vi "rgpna.vi"() -> ()   [LabVIEW 2010]
uses:
  <vilib>/Utility/error.llb/DialogType.ctl
  <vilib>/measure/maspectr.llb/FFT Power Spectrum and PSD for 1 Chan.vi
  <vilib>/Platform/browser.llb/Open URL in Default Browser (string).vi
  user32.dll
  <vilib>/measure/NI_MAPro.lvlib
panel:
  in  "Tab Control":enum32{"View/Edit", "History", "List", "Graph"}(tab)
  in  "String":string
  out "Table":string[][](table)
  in  "Tree":string(tree)
  out "Waveform Graph":cluster{"f0":dbl, "df":dbl, "magnitude":dbl[]}[](graph) caption="-----------------------------------------------------------------------------------"
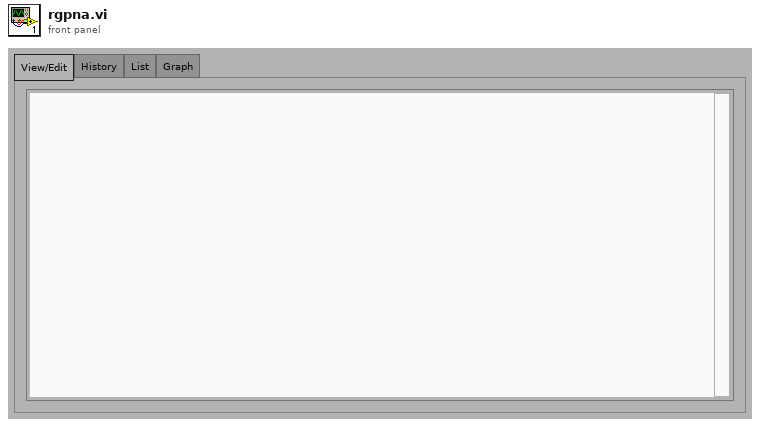
[diagram p1: front panel]
types:
  T1 = typedef "DialogType.ctl" = u16
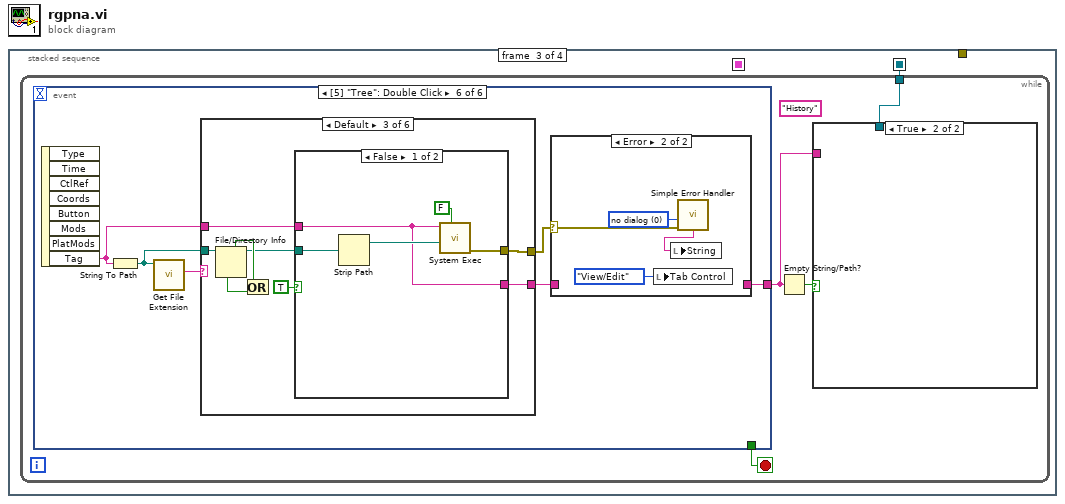
[diagram p0: block diagram]
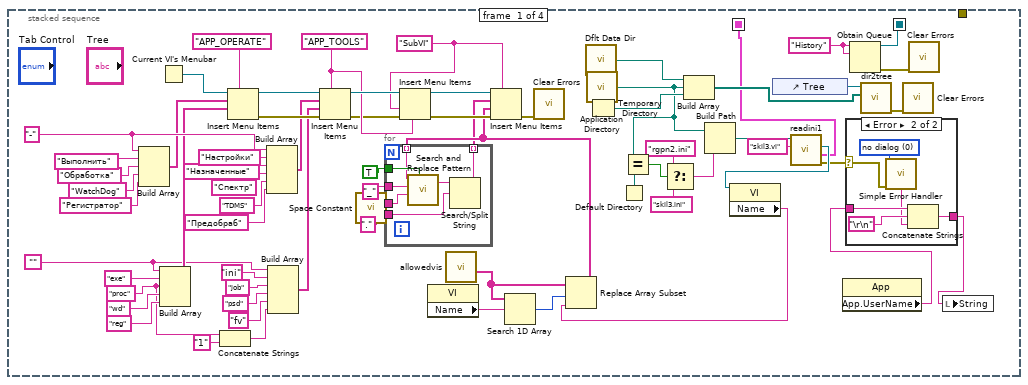
[diagram p2: hidden frame]
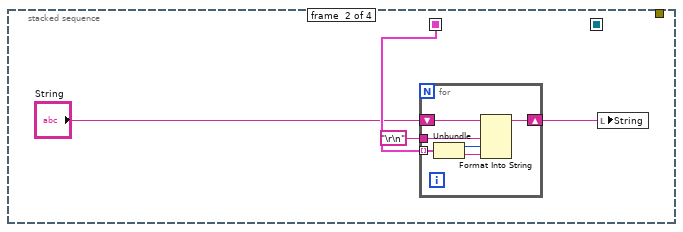
[diagram p4: hidden frame]
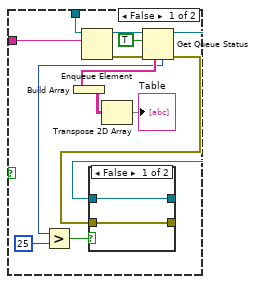
[diagram p5: hidden frame]
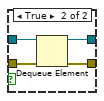
[diagram p6: hidden frame]
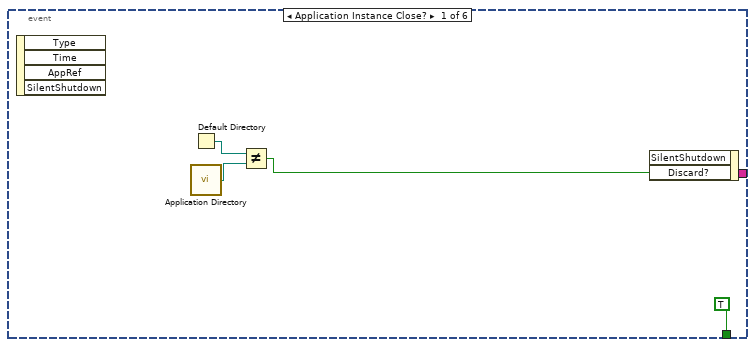
[diagram p7: hidden frame]
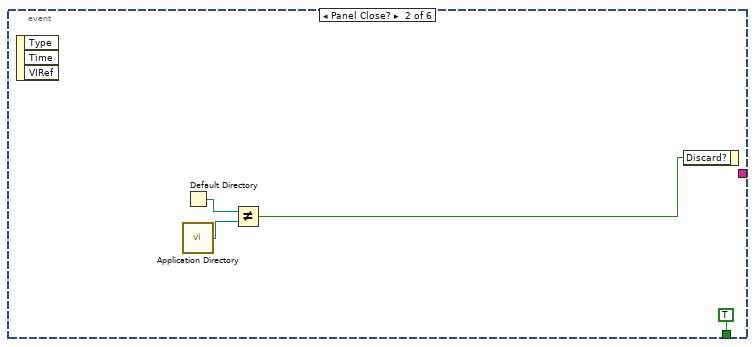
[diagram p8: hidden frame]
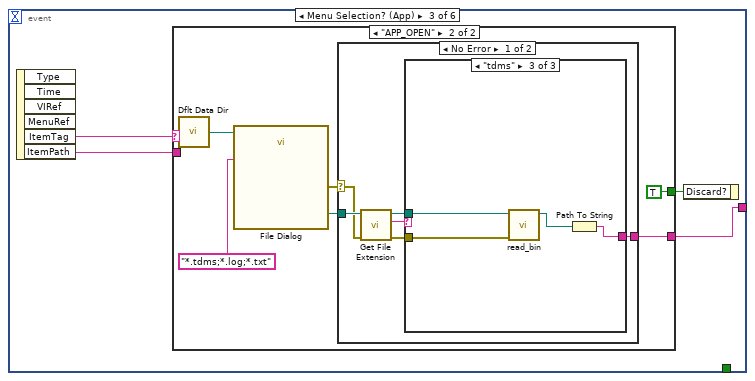
[diagram p9: hidden frame]
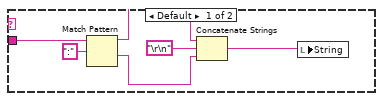
[diagram p10: hidden frame]
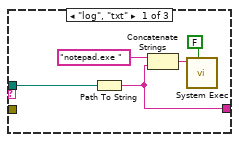
[diagram p11: hidden frame]
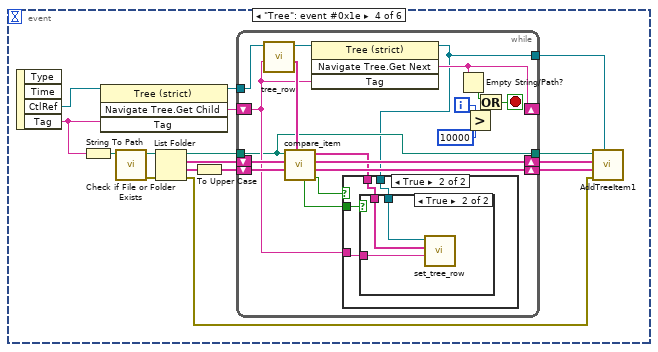
[diagram p14: hidden frame]
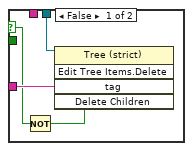
[diagram p15: hidden frame]
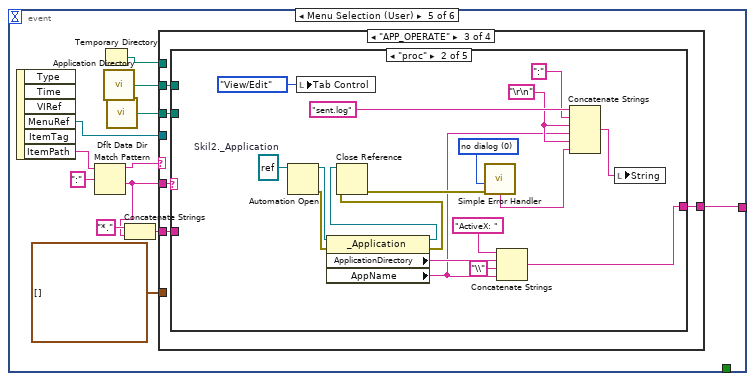
[diagram p17: hidden frame]
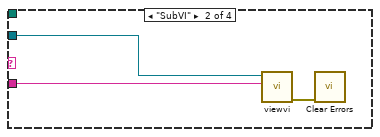
[diagram p19: hidden frame]
diagram:
  n1 = stacked-sequence {
    seq-local: [w51 _ _ _] -> [_ _ w92 w457]
    seq-local: [w13 _ _ _] -> [_ w85 _ _]
    tunnel: [_ _ _ w455] -> _
    frame #0 {
      w43 = "SubVI"
      w3 = "proc" ("element")
      w53 = "History" ("name (unnamed)")
      w54 = ""
      w62 = "-"
      w44 = "APP_TOOLS" ("menu tag")
      n2 = Build Array(w62, "Выполнить", "Обработка", "WatchDog" ("element"), "Регистратор" ("element")) -> (w57:string[])
      n3 = Current VI's Menubar() -> (w67:refnum<k9>)
      n4 = Build Array(w54, "exe", w3, "wd" ("element"), "reg" ("element")) -> (w58:string[])
      n5 = Concatenate Strings(w3, "1" ("string")) -> (w1:string)
      n6 = Insert Menu Items(5:"APP_OPERATE", 7:w58, 8:w57, 9:w67) -> (0:w65:errorcluster, 3:w64:refnum<k9>)  [unwired: 2 in, 1 out]
      n7 = Build Array(w62, "Настройки", "Назначенные" ("element"), "Спектр" ("element"), "TDMS" ("element"), "Предобраб" ("element")) -> (w55:string[])
      n8 = Build Array(w54, "ini", "job" ("element"), "psd" ("element"), "fv" ("element"), w1) -> (w56:string[])
      n9 = Insert Menu Items(5:w44, 6:w65, 7:w56, 8:w55, 9:w64) -> (0:w41:errorcluster, 3:w45:refnum<k9>)  [unwired: 1 in, 1 out]
      n10 = call <vilib>:"Space Constant.vi"() -> ("String"=w15:string)
      n11 = Insert Menu Items(4:w44, 6:w41, 7:w43, 9:w45) -> (0:w40:errorcluster, 3:w42:refnum<k9>)  [unwired: 2 in, 1 out]
      n12 = property class="VI"() -> ("Name"=w29:string)  [unwired: 2 in, 2 out]
      n13 = call "allowedvis.vi"() -> ("AllowedVis"=w38:string[])  [unwired: 6 in, 1 out]
      n14 = Search 1D Array(1D array=w38, element=w29) -> (index of element=w32:i32)  [unwired: 1 in]
      n15 = call <vilib>:"Dflt Data Dir.vi"() -> ("App:Default Data Directory"=w37:path)
      n16 = call <vilib>:"Application Directory.vi"() -> ("Application Directory"=w28:path)
      n17 = Temporary Directory() -> (w36:path)
      n18 = Default Directory() -> (w27:path)
      n19 = Equal?(x=w28, y=w27) -> (x = y?=w26:bool)
      n20 = Select(t="rgpn2.ini" ("name or relative path"), s=w26, f="skil3.ini") -> (s? t:f=w24:string)
      n21 = Build Array(w37, w28, w36) -> (w35:path[])
      n22 = Build Path(base path=w28, name or relative path=w24) -> (appended path=w34:path)
      n23 = control-ref of="Tree"() -> (w52:refnum<vi>)
      n24 = call "readini1.vi"("section"="skil3.vi", "configuration file path"=w34) -> ("error out"=w22:errorcluster, "Dev_Gr"=w13:cluster{"DevNo":i32, "Group":string}[], "global2vi_ref"=w31:refnum<vi>)  [unwired: 2 in, 1 out]
      n25 = property class="VI"(reference=w31) -> ("Name"=w30:string)  [unwired: 1 in, 2 out]
      n26 = Replace Array Subset(array=w38, new element=w30, index=w32) -> (w19:string[])
      n27 = for {
        tunnel: "_" ("regular expression (\"\")") -> [w74]
        tunnel: TRUE ("replace all? (F)") -> [w73]
        tunnel: w19 -> [w72] mode=indexing
        tunnel: [w69] -> w18 mode=indexing
        tunnel: w15 -> [w71]
        tunnel: "." ("regular expression (\"\")") -> [w68]
        n28 = call <vilib>:"Search and Replace Pattern.vi"("string"=w72, "regular expression (\"\")"=w74, "replace string (\"\")"=w71, "replace all? (F)"=w73) -> ("result string"=w70:string)  [unwired: 1 in, 1 out]
        n29 = Search/Split String(string=w70, search string/char (-)=w68) -> (substring before match=w69:string)  [unwired: 1 in, 2 out]
      }
      n30 = Insert Menu Items(5:w43, 6:w40, 7:w19, 8:w18, 9:w42) -> (0:w39:errorcluster)  [unwired: 1 in, 2 out]
      n31 = call <vilib>:"Clear Errors.vi"("error in (no error)"=w39) -> ()  [unwired: 6 in, 1 out]
      n32 = property class="App"() -> ("App.UserName"=w12:string)  [unwired: 2 in, 2 out]
      n33 = case shown="Error" w22 {
        selector: w22 -> [_ w80]
        tunnel: w12 -> [w75 w78]
        tunnel: [w75 w79] -> w11
        frame No Error {
        }
        frame Error {
          w81 = T1 0 items=["no dialog", "OK message", "continue or stop message", "OK message + warnings", "continue/stop + warnings"] ("type of dialog (OK msg:1)")
          n34 = call <vilib>:"Simple Error Handler.vi"("type of dialog (OK msg:1)"=w81, "error in (no error)"=w80) -> ("message"=w76:string)  [unwired: 3 in, 4 out]
          n35 = Concatenate Strings(w78, "\r\n", w76) -> (w79:string)
        }
      }
      n36 = Obtain Queue(name (unnamed)=w53, element data type=w53) -> (queue out=w51:refnum<queue>, error out=w50:errorcluster)  [unwired: 3 in, 1 out]
      n37 = call "dir2tree.vi"("Dirs"=w35, "Tree"=w52) -> ("error out"=w49:errorcluster)  [unwired: 4 in, 1 out]
      n38 = call <vilib>:"Clear Errors.vi"("error in (no error)"=w49) -> ()  [unwired: 6 in, 1 out]
      n39 = call <vilib>:"Clear Errors.vi"("error in (no error)"=w50) -> ()  [unwired: 6 in, 1 out]
      n40 = local write "String"(w11) -> ()
    }
    frame #1 {
      n41 = for {
        tunnel: w85 -> [w91] mode=indexing
        shift-right: [w87] -> w83
        shift-left: "String" -> [w90]
        tunnel: "\r\n" -> [w86]
        n42 = Unbundle(w91) -> ("DevNo"=w89:i32, "Group"=w88:string)
        n43 = Format Into String(initial string=w90, w86, w89, w88) -> (resulting string=w87:string)  [unwired: 2 in, 1 out]
      }
      n44 = local write "String"(w83) -> ()
    }
    frame #2 {
      n45 = while {
        tunnel: w92 -> [w93]
        stop <- w96 stop-if-true
        (unwired) "History" ("name (unnamed)")
        n46 = event shown="[5] \"Tree\": Double Click" {
          selector: _ -> [_ _ _ _ _ _]
          dyn-events: _ -> [_ _ _ _ _ _]
          timeout: _ -> [_ _ _ _ _ _]
          tunnel: [TRUE ("SilentShutdown") TRUE ("SilentShutdown") _ _ _ _] -> w96
          tunnel: [_ _ w124 _ w204 w403] -> w94
          event Application Instance Close? {
            n47 = event-data() -> ()  [unwired: 1 in, 4 out]
            n48 = Default Directory() -> (w119:path)
            n49 = call <vilib>:"Application Directory.vi"() -> ("Application Directory"=w118:path)
            n50 = Not Equal?(x=w119, y=w118) -> (x != y?=w117:bool)
            n51 = event-data("Discard?"=w117) -> ()  [unwired: 2 in, 1 out]
          }
          event Panel Close? {
            n52 = event-data() -> ()  [unwired: 1 in, 3 out]
            n53 = Default Directory() -> (w123:path)
            n54 = call <vilib>:"Application Directory.vi"() -> ("Application Directory"=w122:path)
            n55 = Not Equal?(x=w123, y=w122) -> (x != y?=w121:bool)
            n56 = event-data("Discard?"=w121) -> ()  [unwired: 1 in, 1 out]
          }
          event Menu Selection? (App) {
            n57 = event-data() -> ("ItemTag"=w127:string, "ItemPath"=w125:string)  [unwired: 1 in, 4 out]
            n58 = case shown="\"APP_OPEN\"" w127 {
              tunnel: [_ TRUE ("Discard?")] -> w126
              tunnel: w125 -> [w133 _]
              tunnel: [_ w134] -> w124
              frame Default {
                n59 = Match Pattern(string=w133, regular expression=":") -> (before substring=w131:string, after substring=w130:string)  [unwired: 1 in, 2 out]
                n60 = Concatenate Strings(w131, "\r\n", w130) -> (w128:string)
                n61 = local write "String"(w128) -> ()
              }
              frame "APP_OPEN" {
                n62 = call <vilib>:"Dflt Data Dir.vi"() -> ("App:Default Data Directory"=w138:path)
                n63 = call "File Dialog"("start path"=w138, "pattern (all files)"="*.tdms;*.log;*.txt") -> ("selected path"=w136:path, "error out"=w135:errorcluster)  [unwired: 10 in, 2 out]
                n64 = case shown="No Error" w135 {
                  selector: w135 -> [w141 _]
                  tunnel: w136 -> [w145 _]
                  tunnel: [w140 _] -> w134
                  frame No Error {
                    n65 = call <vilib>:"Get File Extension.vi"("error in (no error)"=w141, "file"=w145) -> ("error out"=w143:errorcluster, "lowercase file extension"=w144:string, "dup file"=w142:path)  [unwired: 6 in, 1 out]
                    n66 = case shown="\"tdms\"" w144 {
                      tunnel: w143 -> [_ _ w154]
                      tunnel: w142 -> [w147 _ w153]
                      tunnel: [w146 _ w151] -> w140
                      frame "log", "txt" {
                        n67 = Path To String(path=w147) -> (string=w146:string)
                        n68 = Concatenate Strings("notepad.exe " ("string"), w146) -> (w149:string)
                        n69 = call <vilib>:"System Exec.vi"("wait until completion? (T)"=FALSE, "command line"=w149) -> ()  [unwired: 6 in, 4 out]
                      }
                      frame Default {
                      }
                      frame "tdms" {
                        n70 = call "read_bin.vi"("error in"=w154, "datalog path"=w153) -> ("new file path"=w152:path)  [unwired: 2 in, 3 out]
                        n71 = Path To String(path=w152) -> (string=w151:string)
                      }
                    }
                  }
                  frame Error {
                  }
                }
              }
            }
            n72 = event-data("Discard?"=w126) -> ()  [unwired: 1 in, 1 out]
          }
          event "Tree": event #0x1e {
            n73 = event-data() -> ("CtlRef"=w170:refnum<vi>, "Tag"=w160:string)  [unwired: 1 in, 2 out]
            n74 = String To Path(string=w160) -> (path=w167:path)
            n75 = invoke class="Tree (strict)" method="Navigate Tree.Get Child"(reference=w170, "Tag"=w160) -> (reference out=w169:refnum<vi>, "Navigate Tree:Get Child"=w168:string)  [unwired: 2 in, 2 out]
            n76 = call <vilib>:"Check if File or Folder Exists.vi"("path"=w167) -> ("error out"=w166:errorcluster, "dup path"=w165:path)  [unwired: 8 in, 1 out]
            n77 = List Folder(path=w165, error in=w166) -> (path out=w163:path, filenames=w162:string[], folder names=w164:string[], error out=w155:errorcluster)  [unwired: 2 in]
            n78 = To Upper Case(1:w164) -> (0:w161:string[])
            n79 = while {
              tunnel: w169 -> [w184]
              tunnel: w163 -> [w172]
              shift-right: [w186] -> w158
              shift-left: w161 -> [w187]
              shift-right: [w185] -> w159
              shift-left: w162 -> [w188]
              shift-right: [w182] -> _
              shift-left: w168 -> [w175]
              tunnel: [w172] -> w157
              tunnel: [w171] -> w156
              i -> [w181]
              stop <- w177 stop-if-true
              n80 = call "tree_row.vi"("Tag"=w175, "CtlRef"=w184) -> ("Row"=w189:string[], "CtlRef 2"=w183:refnum<vi>)  [unwired: 3 in, 1 out]
              n81 = call "compare_item.vi"("item"=w189, "folders"=w187, "filenames"=w188, "start path"=w172) -> ("exist"=w176:bool, "folders 2"=w186:string[], "filenames 2"=w185:string[], "item 2"=w173:string[], "modified"=w174:bool)  [unwired: 1 in]
              n82 = invoke class="Tree (strict)" method="Navigate Tree.Get Next"(reference=w183, "Tag"=w175) -> (reference out=w171:refnum<vi>, "Navigate Tree:Get Next Item"=w182:string)  [unwired: 2 in, 2 out]
              n83 = case shown="True" w176 {
                selector: w176 -> [w190 _]
                tunnel: w171 -> [w193 w196]
                tunnel: w175 -> [w192 w195]
                tunnel: w174 -> [_ w197]
                tunnel: w173 -> [_ w194]
                frame False {
                  n84 = Not(x=w190) -> (.not. x?=w191:bool)
                  n85 = invoke class="Tree (strict)" method="Edit Tree Items.Delete"(reference=w193, "tag"=w192, "Delete Children"=w191) -> ()  [unwired: 2 in, 5 out]
                }
                frame True {
                  n86 = case shown="True" w197 {
                    tunnel: w196 -> [_ w200]
                    tunnel: w195 -> [_ w199]
                    tunnel: w194 -> [_ w198]
                    frame False {
                      # "do nothing"
                    }
                    frame True {
                      n87 = call "set_tree_row.vi"("Tag"=w199, "Row"=w198, "CtlRef"=w200) -> ()  [unwired: 3 in, 2 out]
                    }
                  }
                }
              }
              n88 = Empty String/Path?(string/path=w182) -> (empty?=w179:bool)
              n89 = Greater?(x=w181, y=10000) -> (0:w178:bool)
              n90 = Or(x=w179, y=w178) -> (x .or. y?=w177:bool)
            }
            n91 = call "AddTreeItem1.vi"("CtlRef 2"=w156, "error in"=w155, "folder names"=w158, "filenames"=w159, "path"=w157) -> ()  [unwired: 1 in, 4 out]
          }
          event Menu Selection (User) {
            n92 = event-data() -> ("MenuRef"=w202:refnum<k9>, "ItemPath"=w211:string)  [unwired: 1 in, 4 out]
            n93 = Match Pattern(string=w211, regular expression=":") -> (before substring=w210:string, after substring=w208:string)  [unwired: 1 in, 2 out]
            n94 = Temporary Directory() -> (w205:path)
            n95 = call <vilib>:"Application Directory.vi"() -> ("Application Directory"=w206:path)
            n96 = call <vilib>:"Dflt Data Dir.vi"() -> ("App:Default Data Directory"=w203:path)
            n97 = Concatenate Strings("*." ("string"), w208) -> (w207:string)
            n98 = case shown="\"APP_OPERATE\"" w210 {
              tunnel: w208 -> [_ w215 w220 w302]
              tunnel: w207 -> [_ _ w219 w301]
              tunnel: w206 -> [_ _ w218 w300]
              tunnel: w205 -> [_ _ _ _]
              tunnel: [_ _ w217 w299] -> w204
              tunnel: w203 -> [_ _ w216 w297]
              tunnel: w202 -> [_ w214 _ _]
              tunnel: waveform(i16)[] [] ("Waveform Graph") -> [_ _ _ w298]
              frame Default {
              }
              frame "SubVI" {
                n99 = call "viewvi.vi"("item tag"=w215, "menu reference"=w214) -> ("error out"=w213:errorcluster)  [unwired: 5 in]
                n100 = call <vilib>:"Clear Errors.vi"("error in (no error)"=w213) -> ()  [unwired: 6 in, 1 out]
              }
              frame "APP_OPERATE" {
                n101 = case shown="\"proc\"" w220 {
                  tunnel: w219 -> [_ _ _ w256 _]
                  tunnel: w218 -> [_ _ _ w255 _]
                  tunnel: [_ w228 w246 w254 w264] -> w217
                  tunnel: w216 -> [_ _ _ _ w269]
                  frame Default {
                  }
                  frame "proc" {
                    w232 = "\r\n"
                    w236 = T1 0 items=["no dialog", "OK message", "continue or stop message", "OK message + warnings", "continue/stop + warnings"] ("type of dialog (OK msg:1)")
                    w238 = refnum<k7> refnum  # Skil2._Application
                    n102 = Automation Open(Automation Refnum=w238) -> (Automation Refnum=w230:refnum<k7>, error out=w227:errorcluster)  [unwired: 3 in]
                    n103 = local write "Tab Control"(enum32{"View/Edit", "History", "List", "Graph"}."View/Edit" ("Tab Control")) -> ()
                    n104 = property class="_Application"(reference=w230, error in=w227) -> (reference out=w226:refnum<k7>, error out=w225:errorcluster, "ApplicationDirectory"=w229:string, "AppName"=w221:string)
                    n105 = Close Reference(reference=w226, error in (no error)=w225) -> (error out=w222:errorcluster)
                    n106 = call <vilib>:"Simple Error Handler.vi"("type of dialog (OK msg:1)"=w236, "error in (no error)"=w222) -> ("message"=w231:string)  [unwired: 3 in, 4 out]
                    n107 = Concatenate Strings("ActiveX: " ("string"), w229, "\\" ("string"), w221) -> (w228:string)
                    n108 = Concatenate Strings("sent.log" ("name or relative path"), ":" ("string"), w232, w221, w232, w231) -> (w234:string)
                    n109 = local write "String"(w234) -> ()
                  }
                  frame "reg" {
                    w249 = refnum<k7> refnum  # Rgpn2._Application
                    n110 = Automation Open(Automation Refnum=w249) -> (Automation Refnum=w248:refnum<k7>, error out=w245:errorcluster)  [unwired: 3 in]
                    n111 = property class="_Application"(reference=w248, error in=w245) -> (reference out=w244:refnum<k7>, error out=w243:errorcluster, "ApplicationDirectory"=w247:string, "AppName"=w241:string)
                    n112 = Close Reference(reference=w244, error in (no error)=w243) -> (error out=w239:errorcluster)
                    n113 = case shown="Error" w239 {
                      selector: w239 -> [_ w251]
                      frame No Error {
                      }
                      frame Error {
                        w253 = T1 0 items=["no dialog", "OK message", "continue or stop message", "OK message + warnings", "continue/stop + warnings"] ("type of dialog (OK msg:1)")
                        n114 = call <vilib>:"Simple Error Handler.vi"("type of dialog (OK msg:1)"=w253, "error in (no error)"=w251) -> ("message"=w252:string)  [unwired: 3 in, 4 out]
                        n115 = local write "Tab Control"(enum32{"View/Edit", "History", "List", "Graph"}."View/Edit" ("Tab Control")) -> ()
                        n116 = local write "String"(w252) -> ()
                      }
                    }
                    n117 = Concatenate Strings("ActiveX: " ("string"), w247, "\\" ("string"), w241) -> (w246:string)
                  }
                  frame "exe" {
                    n118 = call "File Dialog2"("start path"=w255, "pattern (all files)"=w256) -> ("selected path"=w257:path, "error out"=w258:errorcluster)  [unwired: 10 in, 2 out]
                    n119 = case shown="No Error" w258 {
                      tunnel: w255 -> [w262 _]
                      tunnel: w257 -> [w261 _]
                      tunnel: [w259 _] -> w254
                      frame No Error {
                        n120 = Path To String(path=w261) -> (string=w259:string)
                        n121 = call <vilib>:"System Exec.vi"("wait until completion? (T)"=FALSE, "working directory"=w262, "command line"=w259) -> ("error out"=w260:errorcluster)  [unwired: 5 in, 3 out]
                        n122 = call <vilib>:"Clear Errors.vi"("error in (no error)"=w260) -> ()  [unwired: 6 in, 1 out]
                      }
                      frame Error {
                      }
                    }
                  }
                  frame "wd" {
                    w267 = "wd.log" ("name or relative path")
                    w264 = "schtasks /run /tn \"watchdog\"" ("command line")
                    n123 = Build Path(base path=w269, name or relative path=w267) -> (appended path=w268:path)
                    n124 = local write "Tab Control"(enum32{"View/Edit", "History", "List", "Graph"}."View/Edit" ("Tab Control")) -> ()
                    n125 = call <vilib>:"System Exec.vi"("run minimized? (F)"=TRUE, "command line"=w264) -> ("error out"=w274:errorcluster, "standard error"=w266:string, "standard output"=w276:string)  [unwired: 6 in, 1 out]
                    n126 = Concatenate Strings(w276, w266) -> (w275:string)
                    n127 = Empty String/Path?(string/path=w266) -> (empty?=w265:bool)
                    n128 = dll-call lib="user32.dll" fn="OemToCharA"(error in=w274, "src"=w275, "dst"=w275) -> (error out=w273:errorcluster, "dst"=w271:string)  [unwired: 4 in, 1 out]
                    n129 = case shown="No Error" w273 {
                      selector: w273 -> [_ w296]
                      tunnel: [w285 w295] -> w272
                      tunnel: w271 -> [w286 _]
                      tunnel: w268 -> [w287 _]
                      tunnel: w267 -> [w280 _]
                      tunnel: w265 -> [w281 _]
                      tunnel: w264 -> [w278 _]
                      frame No Error {
                        w283 = "\r\n"
                        n130 = case shown="True" w281 {
                          tunnel: w287 -> [_ w292]
                          tunnel: [_ w291] -> w282
                          tunnel: [_ w290] -> _
                          tunnel: w280 -> [_ w289]
                          tunnel: [w288 w289] -> w279
                          tunnel: w278 -> [w288 _]
                          frame False {
                          }
                          frame True {
                            n131 = Read from Text File(file (use dialog)=w292) -> (refnum out=w293:refnum<file>, text=w291:string, error out=w294:errorcluster)  [unwired: 3 in, 1 out]
                            n132 = Close File(refnum=w293, error in=w294) -> (error out=w290:errorcluster)  [unwired: 1 out]
                          }
                        }
                        n133 = Concatenate Strings(w286, w283, w279, ":" ("string"), w283, w282) -> (w285:string)
                      }
                      frame Error {
                        n134 = call <vilib>:"Simple Error Handler.vi"("error in (no error)"=w296) -> ("message"=w295:string)  [unwired: 4 in, 4 out]
                      }
                    }
                    n135 = local write "String"(w272) -> ()
                  }
                }
              }
              frame "APP_TOOLS" {
                n136 = case shown="\"proc1\"" w302 {
                  tunnel: w301 -> [_ _ _ w339 _ _]
                  tunnel: w300 -> [_ _ _ w337 _ _]
                  tunnel: [_ w303 w323 w336 w347 _] -> w299
                  tunnel: w298 -> [_ _ _ _ _ w370]
                  tunnel: w297 -> [_ w312 _ _ _ _]
                  frame Default {
                  }
                  frame "proc1" {
                    n137 = Get Date/Time In Seconds() -> (seconds since 1Jan1904=w307:timestamp)
                    n138 = call "File Dialog5"("start path"=w312, "pattern (all files)"="*.tdms") -> ("selected path"=w309:path, "cancelled"=w310:bool)  [unwired: 10 in, 2 out]
                    n139 = To Double Precision Float(number=w307) -> (double precision float=w308:dbl)
                    n140 = call "to_utc.vi"("Numeric"=w308) -> ("Time Stamp"=w306:timestamp)
                    n141 = case shown="False" w310 {
                      tunnel: w309 -> [w322 _]
                      tunnel: w306 -> [w321 _]
                      tunnel: [w320 _] -> w305
                      tunnel: [w319 _] -> w304
                      frame False {
                        n142 = call "poster1.vi"("last ses time"=w321, "file path"=w322) -> ("error out"=w320:errorcluster, "file dup"=w319:path)  [unwired: 3 in, 1 out]
                      }
                      frame True {
                      }
                    }
                    n143 = case shown="Error" w305 {
                      selector: w305 -> [_ w318]
                      tunnel: w304 -> [w314 _]
                      tunnel: [w313 _] -> w303
                      frame No Error {
                        n144 = Path To String(path=w314) -> (string=w313:string)
                      }
                      frame Error {
                        w317 = T1 0 items=["no dialog", "OK message", "continue or stop message", "OK message + warnings", "continue/stop + warnings"] ("type of dialog (OK msg:1)")
                        n145 = call <vilib>:"Simple Error Handler.vi"("type of dialog (OK msg:1)"=w317, "error in (no error)"=w318) -> ("message"=w316:string)  [unwired: 3 in, 4 out]
                        n146 = local write "Tab Control"(enum32{"View/Edit", "History", "List", "Graph"}."View/Edit" ("Tab Control")) -> ()
                        n147 = local write "String"(w316) -> ()
                      }
                    }
                  }
                  frame "fv" {
                    n148 = call <vilib>:"Dflt Data Dir.vi"() -> ("App:Default Data Directory"=w325:path)
                    n149 = Build Path(base path=w325, name or relative path="Sent") -> (appended path=w324:path)
                    n150 = call "File Dialog4"("start path"=w324, "pattern (all files)"="*.tdms") -> ("selected path"=w330:path, "cancelled"=w327:bool, "error out"=w329:errorcluster)  [unwired: 10 in, 1 out]
                    n151 = case shown="False" w327 {
                      tunnel: [w335 _] -> _
                      tunnel: w330 -> [w334 _]
                      tunnel: w329 -> [w333 _]
                      tunnel: [w331 _] -> w323
                      frame False {
                        n152 = call <vilib>:"TDMS - File Viewer.vi"("error in (no error)"=w333, "file path"=w334) -> ("error out"=w335:errorcluster, "file path out"=w332:path)  [unwired: 4 in]
                        n153 = Path To String(path=w332) -> (string=w331:string)
                      }
                      frame True {
                      }
                    }
                  }
                  frame "ini" {
                    n154 = call "File Dialog3"("start path"=w337, "pattern (all files)"=w339) -> ("selected path"=w338:path, "error out"=w340:errorcluster)  [unwired: 10 in, 2 out]
                    n155 = case shown="No Error" w340 {
                      tunnel: w338 -> [w342 _]
                      tunnel: [w341 _] -> w336
                      frame No Error {
                        n156 = Path To String(path=w342) -> (string=w341:string)
                        n157 = Concatenate Strings("notepad.exe " ("string"), w341) -> (w345:string)
                        n158 = call <vilib>:"System Exec.vi"("wait until completion? (T)"=FALSE, "command line"=w345) -> ("error out"=w343:errorcluster)  [unwired: 6 in, 3 out]
                        n159 = call <vilib>:"Clear Errors.vi"("error in (no error)"=w343) -> ()  [unwired: 6 in, 1 out]
                      }
                      frame Error {
                      }
                    }
                  }
                  frame "job" {
                    (unwired) " /tn watchdog"
                    w347 = "schtasks /query"
                    n160 = call <vilib>:"System Exec.vi"("run minimized? (F)"=TRUE, "command line"=w347) -> ("error out"=w353:errorcluster, "standard error"=w355:string, "standard output"=w356:string)  [unwired: 6 in, 1 out]
                    n161 = local write "Tab Control"(enum32{"View/Edit", "History", "List", "Graph"}."View/Edit" ("Tab Control")) -> ()
                    n162 = Concatenate Strings(w356, w355) -> (w352:string)
                    n163 = dll-call lib="user32.dll" fn="OemToCharA"(error in=w353, "src"=w352, "dst"=w352) -> (error out=w351:errorcluster, "dst"=w350:string)  [unwired: 4 in, 1 out]
                    n164 = case shown="Error" w351 {
                      selector: w351 -> [_ w360]
                      tunnel: [w357 w358] -> w348
                      tunnel: w350 -> [w357 _]
                      frame No Error {
                      }
                      frame Error {
                        w359 = T1 0 items=["no dialog", "OK message", "continue or stop message", "OK message + warnings", "continue/stop + warnings"] ("type of dialog (OK msg:1)")
                        n165 = call <vilib>:"Simple Error Handler.vi"("type of dialog (OK msg:1)"=w359, "error in (no error)"=w360) -> ("message"=w358:string)  [unwired: 3 in, 4 out]
                      }
                    }
                    n166 = local write "String"(w348) -> ()
                  }
                  frame "psd" {
                    n167 = Open VI Reference(vi path="read_bin.vi") -> (vi reference=w381:refnum<vi>, error out=w380:errorcluster)  [unwired: 5 in]
                    n168 = invoke class="VI" method="Ctrl Val.Get"(reference=w381, error in=w380, "Control Name"="Waveform Graph") -> (reference out=w375:refnum<vi>, error out=w377:errorcluster, "Get Control Value Variant"=w378:variant)  [unwired: 1 in, 1 out]
                    n169 = property on="Waveform Graph" class="WFGraph (strict)"("XScale.NameLbl.Text"="Freq" ("X Scale.Name Label.Text"), "YScale.NameLbl.Text"="Mag" ("Y Scale.Name Label.Text"), "XScale.Mapping Mode"=u8 1 ("X Scale.Mapping Mode")) -> ()  [unwired: 2 in, 2 out]
                    n170 = Variant To Data(error in=w377, Variant=w378, type=w370) -> (error out=w365:errorcluster, data=w368:waveform(i16)[])
                    n171 = call "split3.vi"("Array of Waveform In"=w368) -> ("Array of Waveform"=w367:waveform(i16)[])  [unwired: 5 in, 1 out]
                    n172 = Close Reference(reference=w375, error in (no error)=w365) -> (error out=w364:errorcluster)
                    n173 = for {
                      tunnel: w367 -> [w392] mode=indexing
                      tunnel: [w390] -> w366 mode=indexing
                      tunnel: w364 -> [w385]
                      tunnel: [w384] -> w363 mode=indexing
                      i -> [w395]
                      n174 = property on="Waveform Graph" class="WFGraph (strict)"(error in=w385, "Active Plot"=w395) -> (error out=w389:errorcluster, "Plot.Plot Name"=w394:string)  [unwired: 1 in, 1 out]
                      n175 = Get Waveform Attribute(4:w389, 5:w394, 6:"NI_ChannelName", 7:w392) -> (0:w388:errorcluster, 1:w393:string, 3:w396:waveform(i16))  [unwired: 1 out]
                      n176 = property on="Waveform Graph" class="WFGraph (strict)"(error in=w388, "Plot.Plot Name"=w393) -> (error out=w387:errorcluster)  [unwired: 1 in, 1 out]
                      n177 = call "mv2v.vi"("y"=5, "WaveformIn"=w396) -> ("Waveform"=w391:waveform(dbl))  [unwired: 5 in]
                      n178 = call-poly <vilib>:"FFT Power Spectrum and PSD.vi"("error in (no error)"=w387, "time signal"=w391) -> ("error out"=w384:errorcluster, "Power Spectrum / PSD"=w390:cluster{"f0":dbl, "df":dbl, "magnitude":dbl[]})  [unwired: 6 in, 2 out]
                      n179 = Wait (ms)(milliseconds to wait=u32 11) -> ()  [unwired: 1 out]
                    }
                    n180 = control-ref of="Waveform Graph"() -> (w369:refnum<vi>)
                    n181 = Merge Errors(w363) -> (w362:errorcluster)
                    n182 = call "3phColor.vi"("error in (no error)"=w362, "Waveform Graph"=w369) -> ("error out"=w361:errorcluster)  [unwired: 5 in]
                    n183 = case shown="Error" w361 {
                      selector: w361 -> [_ w401]
                      tunnel: w366 -> [w398 _]
                      tunnel: [enum32{"View/Edit", "History", "List", "Graph"}."Graph" ("Tab Control") enum32{"View/Edit", "History", "List", "Graph"}."View/Edit" ("Tab Control")] -> w376
                      frame No Error {
                        "Waveform Graph" <- w398
                      }
                      frame Error {
                        w400 = T1 0 items=["no dialog", "OK message", "continue or stop message", "OK message + warnings", "continue/stop + warnings"] ("type of dialog (OK msg:1)")
                        n184 = call <vilib>:"Simple Error Handler.vi"("type of dialog (OK msg:1)"=w400, "error in (no error)"=w401) -> ("message"=w399:string)  [unwired: 3 in, 4 out]
                        n185 = local write "String"(w399) -> ()
                      }
                    }
                    n186 = local write "Tab Control"(w376) -> ()
                  }
                }
              }
            }
          }
          event "Tree": Double Click {
            n187 = event-data() -> ("Tag"=w407:string)  [unwired: 1 in, 7 out]
            n188 = String To Path(string=w407) -> (path=w406:path)
            n189 = call <vilib>:"Get File Extension.vi"("file"=w406) -> ("lowercase file extension"=w408:string)  [unwired: 7 in, 3 out]
            n190 = case shown="Default" w408 {
              tunnel: w407 -> [w416 w419 w425 w436 w439 w448]
              tunnel: [_ w420 w423 w436 w439 w448] -> w404
              tunnel: w406 -> [w415 _ w429 w437 w443 _]
              tunnel: [w418 w421 w424 w435 w440 w447] -> w405
              frame "cmd", "exe", "vbs" {
                n191 = Strip Path(path=w415) -> (stripped path=w414:path)  [unwired: 1 out]
                n192 = call <vilib>:"System Exec.vi"("wait until completion? (T)"=FALSE, "working directory"=w414, "command line"=w416) -> ("error out"=w418:errorcluster)  [unwired: 5 in, 3 out]
              }
              frame "htm" {
                n193 = call-poly <vilib>:"Open URL in Default Browser.vi"("URL"=w419) -> ("error out"=w421:errorcluster, "URL out"=w420:string)  [unwired: 5 in]
              }
              frame Default {
                n194 = File/Directory Info(path=w429) -> (path out=w426:path, directory=w428:bool, shortcut=w427:bool)  [unwired: 1 in, 4 out]
                n195 = Or(x=w428, y=w427) -> ()  [unwired: 1 out]
                n196 = case shown="False" TRUE {
                  tunnel: w426 -> [w434 _]
                  tunnel: w425 -> [w430 _]
                  tunnel: [w431 _] -> w424
                  tunnel: [w430 _] -> w423
                  frame False {
                    n197 = Strip Path(path=w434) -> (stripped path=w433:path)  [unwired: 1 out]
                    n198 = call <vilib>:"System Exec.vi"("wait until completion? (T)"=FALSE, "working directory"=w433, "command line"=w430) -> ("error out"=w431:errorcluster)  [unwired: 5 in, 3 out]
                  }
                  frame True {
                  }
                }
              }
              frame "tdms" {
                n199 = call "read_bin.vi"("datalog path"=w437) -> ("error out"=w435:errorcluster)  [unwired: 3 in, 3 out]
              }
              frame "dat" {
                n200 = call "convert_dat2tdms.vi"("temporary?"=TRUE, "Path"=w443) -> ("error out"=w438:errorcluster, "New Filel Path"=w441:path)  [unwired: 4 in]
                n201 = case shown="No Error" w438 {
                  selector: w438 -> [_ w446]
                  tunnel: w441 -> [w445 _]
                  tunnel: [w444 w446] -> w440
                  frame No Error {
                    n202 = call "read_bin.vi"("datalog path"=w445) -> ("error out"=w444:errorcluster)  [unwired: 3 in, 3 out]
                  }
                  frame Error {
                  }
                }
              }
              frame "ini", "log", "txt" {
                n203 = Concatenate Strings("notepad.exe " ("string"), w448) -> (w450:string)
                n204 = call <vilib>:"System Exec.vi"("wait until completion? (T)"=FALSE, "command line"=w450) -> ("error out"=w447:errorcluster)  [unwired: 6 in, 3 out]
              }
            }
            n205 = case shown="Error" w405 {
              selector: w405 -> [_ w410]
              tunnel: w404 -> [w409 _]
              tunnel: [w409 _] -> w403
              frame No Error {
              }
              frame Error {
                w413 = T1 0 items=["no dialog", "OK message", "continue or stop message", "OK message + warnings", "continue/stop + warnings"] ("type of dialog (OK msg:1)")
                n206 = local write "Tab Control"(enum32{"View/Edit", "History", "List", "Graph"}."View/Edit" ("Tab Control")) -> ()
                n207 = call <vilib>:"Simple Error Handler.vi"("type of dialog (OK msg:1)"=w413, "error in (no error)"=w410) -> ("message"=w412:string)  [unwired: 3 in, 4 out]
                n208 = local write "String"(w412) -> ()
              }
            }
          }
        }
        n209 = Empty String/Path?(string/path=w94) -> (empty?=w95:bool)
        n210 = case shown="True" w95 {
          tunnel: w94 -> [w106 _]
          tunnel: w93 -> [w98 _]
          frame False {
            n211 = Enqueue Element(queue=w98, element=w106) -> (queue out=w105:refnum<queue>, error out=w104:errorcluster)  [unwired: 2 in, 1 out]
            n212 = Get Queue Status(queue=w105, return elements? (F)=TRUE, error in (no error)=w104) -> (queue out=w100:refnum<queue>, error out=w99:errorcluster, # elements in queue=w102:i32, elements=w108:string[])  [unwired: 4 out]
            n213 = Greater?(x=w102, y=25) -> (0:w103:bool)
            n214 = Build Array(w108) -> (w107:string[][])
            n215 = case shown="False" w103 {
              tunnel: [w111 w115] -> _
              tunnel: [w110 w114] -> _
              tunnel: w100 -> [w111 w113]
              tunnel: w99 -> [w110 w112]
              frame False {
              }
              frame True {
                n216 = Dequeue Element(queue=w113, error in (no error)=w112) -> (queue out=w115:refnum<queue>, error out=w114:errorcluster)  [unwired: 1 in, 2 out]
              }
            }
            n217 = Transpose 2D Array(2D array=w107) -> (transposed array=→"Table":string[][])
          }
          frame True {
          }
        }
      }
    }
    frame #3 {
      n218 = call <vilib>:"Application Directory.vi"() -> ("Application Directory"=w454:path)
      n219 = Default Directory() -> (w453:path)
      n220 = Equal?(x=w454, y=w453) -> (x = y?=w452:bool)
      n221 = Quit LabVIEW(quit? (T)=w452) -> ()
      n222 = Release Queue(queue=w457, force destroy? (F)=TRUE) -> (error out=w455:errorcluster)  [unwired: 1 in, 2 out]
    }
  }
